vi "Fire Trigger.vi"(10 "Exceed Action":string) -> ()   [LabVIEW 2015]
uses:
  Sequence Global Action.ctl
  Test Control Command.ctl
  System State.ctl
  System State Global Action.ctl
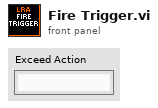
[diagram p1: front panel]
types:
  T1 = typedef "Sequence Global Action.ctl" = enum16{"Get", "Set List", "Set Current"}
  T2 = typedef "Single Test Sequence.ctl" = cluster{"Actions":T3[], "Triggers":T6[], "Name":string}
  T3 = typedef "Test Sequence Action.ctl" = cluster{"Time":i32, "Action":T4, "Valve":T5}
  T4 = typedef "Valve Action Enum.ctl" = enum16{"Open", "Close"}
  T5 = typedef "Valve Name Enum.ctl" = enum16{"FV-2", "FV-3", "FV-4", "OV-2", "OV-3", "OV-4", "NV-2", "COMP"}
  T6 = typedef "Test Sequence Trigger.ctl" = cluster{"Sensor":T7, "Begin Time (ms)":u32, "End Time(ms)":u32, "Min Value":dbl, "Max Value":dbl, "Exceed Action":string}
  T7 = typedef "Sensor Enum.ctl" = enum16{"FPD-1", "FPD-2", "FPD-3", "OPD-1", "OPD-2", "OPD-3", "AP-1", "PC-1", "PC-2", "VBAT", "VCOMP", "ICOMP", "TC-1", "TC-COMP"}
  T8 = typedef "System State Global Action.ctl" = enum16{"Get", "Set", "Initialize"}
  T9 = typedef "System State.ctl" = enum16{"Disabled", "E-Stop", "Standby", "Active"}
  T10 = typedef "Test Control Command.ctl" = enum16{"Get Notifier", "Init", "Start", "Stop"}
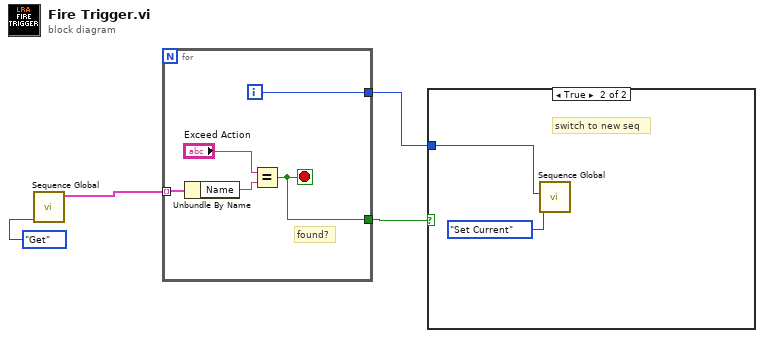
[diagram p0: block diagram]
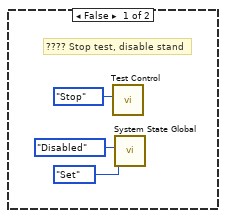
[diagram p2: hidden frame]
diagram:
  n1 = call "Sequence Global.vi"("Action"=Sequence_Global_Action."Get") -> ("Sequence List Out"=w3:T2[])  [unwired: 8 in, 2 out]
  n2 = for {
    tunnel: w3 -> [w9] mode=indexing
    tunnel: [w6] -> w1
    tunnel: [w5] -> w2
    i -> [w6]
    stop <- w5 stop-if-true
    # "found?"
    n3 = Unbundle By Name(w9) -> ("Name"=w8:string)
    n4 = Equal?(x="Exceed Action", y=w8) -> (x = y?=w5:bool)
  }
  n5 = case shown="True" w2 {
    tunnel: w1 -> [_ w13]
    frame False {
      # "???? Stop test, disable stand"
      n6 = call "Test Control.vi"("Command"=Test_Control_Command."Stop") -> ()  [unwired: 10 in, 1 out]
      n7 = call "System State Global.vi"("Action"=System_State_Global_Action."Set", "State In"=System_State."Disabled") -> ()  [unwired: 8 in, 2 out]
    }
    frame True {
      # "switch to new seq"
      n8 = call "Sequence Global.vi"("Action"=Sequence_Global_Action."Set Current", "New Seq Index"=w13) -> ()  [unwired: 7 in, 3 out]
    }
  }
